vi "Delete Message Template Files.vi"(8 "error in (no error)":errorcluster, 11 "LVClassLibrary in":refnum<vi>) -> (0 "error out":errorcluster, 3 "LVClassLibrary out":refnum<vi>)   [LabVIEW 2019, in "gRPC Scripting Tools.lvlib"]
uses:
  gRPC Scripting Tools.lvlib
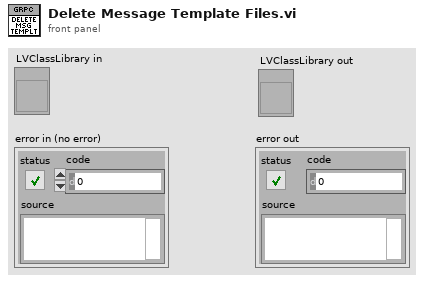
[diagram p1: front panel]
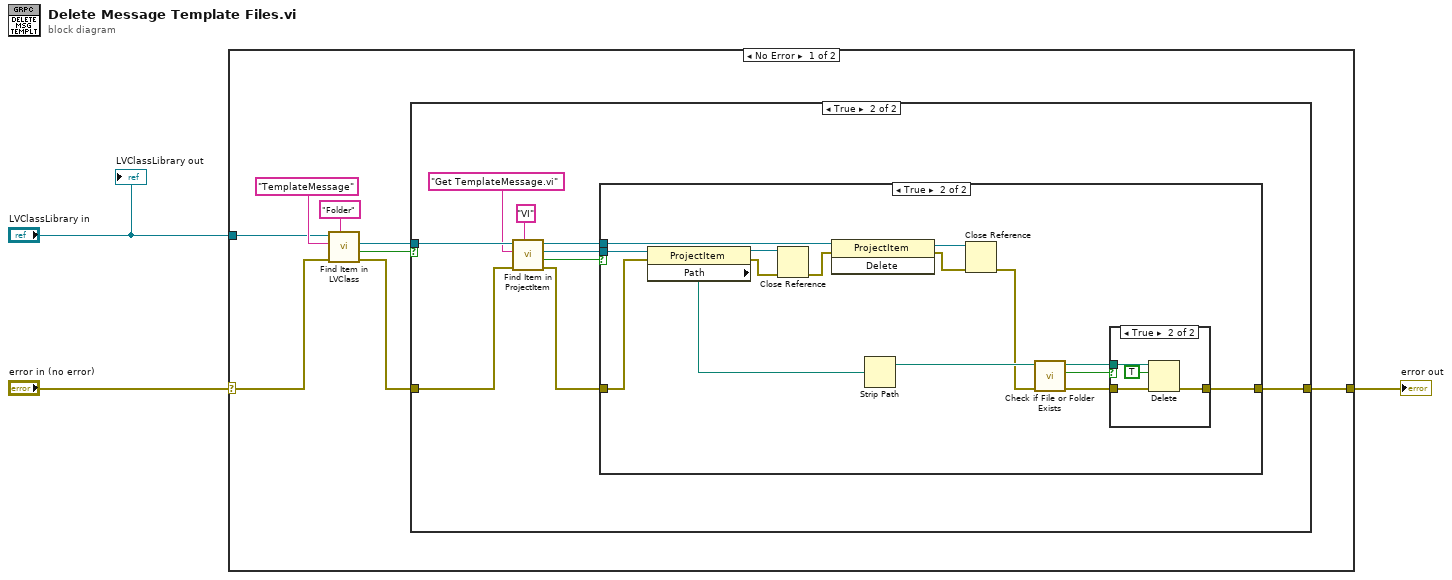
[diagram p0: block diagram]
diagram:
  n1 = case shown="No Error" "error in (no error)" {
    selector: "error in (no error)" -> [w5 w43]
    tunnel: "LVClassLibrary in" -> [w9 _]
    tunnel: [w4 w43] -> w1
    frame No Error {
      n2 = call "Find Item in LVClass.vi"("Item Type"="Folder", "error in (no error)"=w5, "Item Name"="TemplateMessage", "Class Item in"=w9) -> ("error out"=w7:errorcluster, "Found?"=w6:bool, "Project Item (Class Item)"=w8:refnum<vi>)  [unwired: 4 in, 1 out]
      n3 = case shown="True" w6 {
        tunnel: w8 -> [_ w21]
        tunnel: w7 -> [w12 w15]
        tunnel: [w12 w13] -> w4
        frame False {
        }
        frame True {
          n4 = call "Find Item in ProjectItem.vi"("Item Type"="VI", "error in (no error)"=w15, "Name"="Get TemplateMessage.vi" ("Item Type"), "ProjectItem in"=w21) -> ("error out"=w14:errorcluster, "Found ?"=w18:bool, "Item Refnum out"=w16:refnum<vi>, "ProjectItem out"=w17:refnum<vi>)  [unwired: 4 in]
          n5 = case shown="True" w18 {
            tunnel: w14 -> [w22 w37]
            tunnel: w16 -> [_ w36]
            tunnel: w17 -> [_ w31]
            tunnel: [w22 w29] -> w13
            frame False {
            }
            frame True {
              n6 = property class="ProjectItem"(reference=w36, error in=w37) -> (reference out=w28:refnum<vi>, error out=w27:errorcluster, "Path"=w30:path)
              n7 = Close Reference(reference=w28, error in (no error)=w27) -> (error out=w26:errorcluster)
              n8 = invoke class="ProjectItem" method="Delete"(reference=w31, error in=w26) -> (reference out=w24:refnum<vi>, error out=w25:errorcluster)  [unwired: 1 in, 1 out]
              n9 = Strip Path(path=w30) -> (stripped path=w32:path)  [unwired: 1 out]
              n10 = Close Reference(reference=w24, error in (no error)=w25) -> (error out=w23:errorcluster)
              n11 = call <vilib>:"Check if File or Folder Exists.vi"("error in (no error)"=w23, "path"=w32) -> ("error out"=w35:errorcluster, "file or folder exists?"=w33:bool, "dup path"=w34:path)  [unwired: 7 in]
              n12 = case shown="True" w33 {
                tunnel: w34 -> [_ w42]
                tunnel: w35 -> [w38 w41]
                tunnel: [w38 w40] -> w29
                frame False {
                }
                frame True {
                  n13 = Delete(path (use dialog)=w42, entire hierarchy (F)=TRUE, error in=w41) -> (error out=w40:errorcluster)  [unwired: 2 in, 2 out]
                }
              }
            }
          }
        }
      }
    }
    frame Error {
    }
  }
  "error out" <- w1
  "LVClassLibrary out" <- "LVClassLibrary in"
